vi "SimpleWaitABit.vi"(11 "Numeric":dbl) -> (3 "msoutput":dbl)   [LabVIEW 2012]
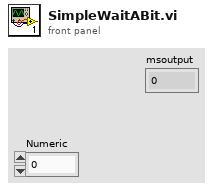
[diagram p1: front panel]
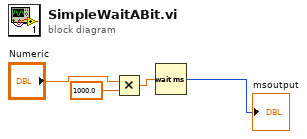
[diagram p0: block diagram]
diagram:
  n1 = Multiply(x="Numeric", y=1000.0) -> (x*y=w2:dbl)
  n2 = Wait (ms)(milliseconds to wait=w2) -> (millisecond timer value=→"msoutput":u32)
